vi "plots_control.vi"(4 "seconds":dbl, 5 "log? plot?":bool, 6 "minutes":dbl, 7 "is first loop?":bool, 8 "capacity":dbl, 9 "temperature":dbl, 10 "current":dbl, 11 "voltage":dbl) -> (0 "capacity cluster":cluster{dbl[], dbl[]}, 1 "temperature cluster":cluster{dbl[], dbl[]}, 2 "current cluster":cluster{dbl[], dbl[]}, 3 "voltage cluster":cluster{dbl[], dbl[]})   [LabVIEW 2016]
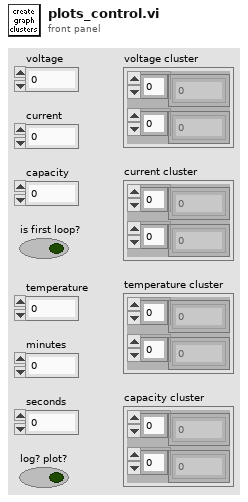
[diagram p1: front panel]
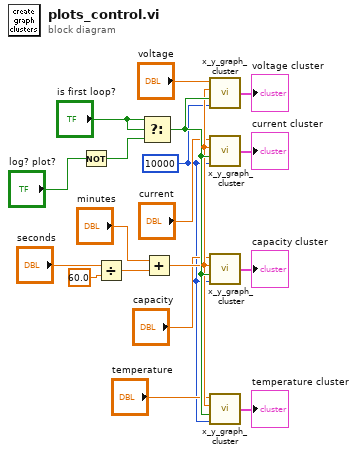
[diagram p0: block diagram]
diagram:
  w5 = 10000 ("Chart History (10,000)")
  n1 = Not(x="log? plot?") -> (.not. x?=w17:bool)
  n2 = Divide(x="seconds", y=60.0) -> (x/y=w9:dbl)
  n3 = Select(t="is first loop?", s="is first loop?", f=w17) -> (s? t:f=w16:bool)
  n4 = Add(x="minutes", y=w9) -> (x+y=w14:dbl)
  n5 = call "x_y_graph_cluster.vi"("Chart History (10,000)"=w5, "Clear Graph?"=w16, "X"=w14, "Y"="voltage") -> ("Cluster"=→"voltage cluster":cluster{dbl[], dbl[]})
  n6 = call "x_y_graph_cluster.vi"("Chart History (10,000)"=w5, "Clear Graph?"=w16, "X"=w14, "Y"="current") -> ("Cluster"=→"current cluster":cluster{dbl[], dbl[]})
  n7 = call "x_y_graph_cluster.vi"("Chart History (10,000)"=w5, "Clear Graph?"=w16, "X"=w14, "Y"="capacity") -> ("Cluster"=→"capacity cluster":cluster{dbl[], dbl[]})
  n8 = call "x_y_graph_cluster.vi"("Chart History (10,000)"=w5, "Clear Graph?"=w16, "X"=w14, "Y"="temperature") -> ("Cluster"=→"temperature cluster":cluster{dbl[], dbl[]})
